vi "Reorder Array__ogtk.vi"   [LabVIEW 2018]
doc: "This polymorphic VI reorders 1D and 2D arrays of any size based on the sorted pointers you specify. For 2D arrays, it reorders by row or by column.\n\n<B>THIS VI IS DEPRICATED</B>. Please use \"Reorder Array2\" (or newer version), available as \"Reorder Array\" from the Functions palette."
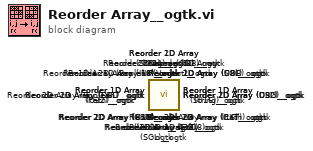
[diagram p0: block diagram]
diagram:
  n1 = call <userlib>:"Reorder 2D Array (Variant)__ogtk.vi"() -> ()  [unwired: 9 in, 3 out]
  n2 = call <userlib>:"Reorder 1D Array (Variant)__ogtk.vi"() -> ()  [unwired: 10 in, 2 out]
  n3 = call <userlib>:"Reorder 1D Array (Path)__ogtk.vi"() -> ()  [unwired: 10 in, 2 out]
  n4 = call <userlib>:"Reorder 1D Array (String)__ogtk.vi"() -> ()  [unwired: 10 in, 2 out]
  n5 = call <userlib>:"Reorder 1D Array (Boolean)__ogtk.vi"() -> ()  [unwired: 10 in, 2 out]
  n6 = call <userlib>:"Reorder 2D Array (Path)__ogtk.vi"() -> ()  [unwired: 9 in, 3 out]
  n7 = call <userlib>:"Reorder 2D Array (String)__ogtk.vi"() -> ()  [unwired: 9 in, 3 out]
  n8 = call <userlib>:"Reorder 2D Array (Boolean)__ogtk.vi"() -> ()  [unwired: 9 in, 3 out]
  n9 = call <userlib>:"Reorder 2D Array (U8)__ogtk.vi"() -> ()  [unwired: 9 in, 3 out]
  n10 = call <userlib>:"Reorder 2D Array (U32)__ogtk.vi"() -> ()  [unwired: 9 in, 3 out]
  n11 = call <userlib>:"Reorder 2D Array (U16)__ogtk.vi"() -> ()  [unwired: 9 in, 3 out]
  n12 = call <userlib>:"Reorder 2D Array (SGL)__ogtk.vi"() -> ()  [unwired: 9 in, 3 out]
  n13 = call <userlib>:"Reorder 2D Array (I8)__ogtk.vi"() -> ()  [unwired: 9 in, 3 out]
  n14 = call <userlib>:"Reorder 2D Array (I32)__ogtk.vi"() -> ()  [unwired: 9 in, 3 out]
  n15 = call <userlib>:"Reorder 2D Array (I16)__ogtk.vi"() -> ()  [unwired: 9 in, 3 out]
  n16 = call <userlib>:"Reorder 2D Array (EXT)__ogtk.vi"() -> ()  [unwired: 9 in, 3 out]
  n17 = call <userlib>:"Reorder 2D Array (DBL)__ogtk.vi"() -> ()  [unwired: 9 in, 3 out]
  n18 = call <userlib>:"Reorder 2D Array (CSG)__ogtk.vi"() -> ()  [unwired: 9 in, 3 out]
  n19 = call <userlib>:"Reorder 2D Array (CXT)__ogtk.vi"() -> ()  [unwired: 9 in, 3 out]
  n20 = call <userlib>:"Reorder 2D Array (CDB)__ogtk.vi"() -> ()  [unwired: 9 in, 3 out]
  n21 = call <userlib>:"Reorder 1D Array (U8)__ogtk.vi"() -> ()  [unwired: 10 in, 2 out]
  n22 = call <userlib>:"Reorder 1D Array (U32)__ogtk.vi"() -> ()  [unwired: 10 in, 2 out]
  n23 = call <userlib>:"Reorder 1D Array (U16)__ogtk.vi"() -> ()  [unwired: 10 in, 2 out]
  n24 = call <userlib>:"Reorder 1D Array (SGL)__ogtk.vi"() -> ()  [unwired: 10 in, 2 out]
  n25 = call <userlib>:"Reorder 1D Array (I8)__ogtk.vi"() -> ()  [unwired: 10 in, 2 out]
  n26 = call <userlib>:"Reorder 1D Array (I32)__ogtk.vi"() -> ()  [unwired: 10 in, 2 out]
  n27 = call <userlib>:"Reorder 1D Array (I16)__ogtk.vi"() -> ()  [unwired: 10 in, 2 out]
  n28 = call <userlib>:"Reorder 1D Array (EXT)__ogtk.vi"() -> ()  [unwired: 10 in, 2 out]
  n29 = call <userlib>:"Reorder 1D Array (DBL)__ogtk.vi"() -> ()  [unwired: 10 in, 2 out]
  n30 = call <userlib>:"Reorder 1D Array (CSG)__ogtk.vi"() -> ()  [unwired: 10 in, 2 out]
  n31 = call <userlib>:"Reorder 1D Array (CXT)__ogtk.vi"() -> ()  [unwired: 10 in, 2 out]
  n32 = call <userlib>:"Reorder 1D Array (CDB)__ogtk.vi"() -> ()  [unwired: 10 in, 2 out]
